vi "Remove Name-UserEvent.vi"(10 "Name":string, 11 "UserEventTimer in":refnum<class "TimerEngine.lvclass">) -> (3 "UserEventTimer out":refnum<class "TimerEngine.lvclass">)   [LabVIEW 2017, in "TimerEngine.lvlib" / "TimerEngine.lvclass"]
uses:
  TimerEngine.lvclass
  TimerEngine.lvclass/TimerEngine.ctl
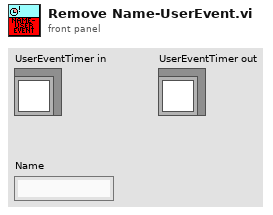
[diagram p1: front panel]
types:
  T1 = typedef "TimerEngine.lvlib/TimerEngine.lvclass/Timer-Userevent.ctl" = refnum<user-event>
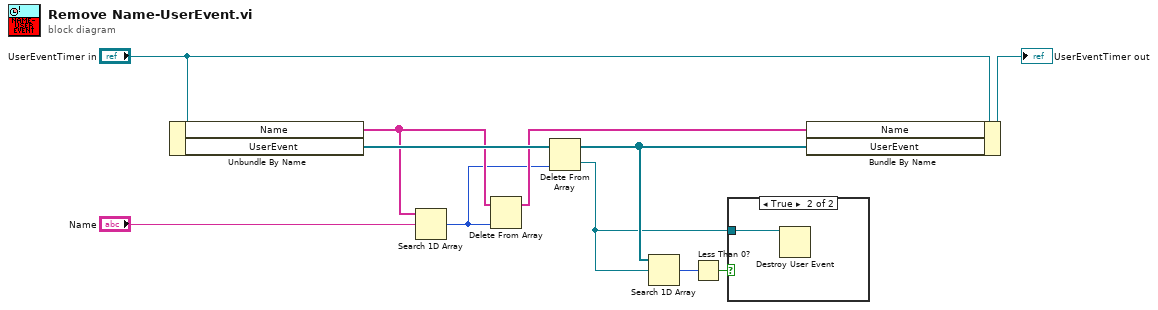
[diagram p0: block diagram]
diagram:
  n1 = Unbundle By Name("UserEventTimer in") -> ("Name"=w7:string[], "UserEvent"=w9:T1[])
  n2 = Search 1D Array(1D array=w7, element="Name") -> (index of element=w5:i32)  [unwired: 1 in]
  n3 = Delete From Array(array=w7, index=w5) -> (array with subset deleted=w6:string[])  [unwired: 1 in, 1 out]
  n4 = Delete From Array(array=w9, index=w5) -> (deleted portion=w2:T1, array with subset deleted=w4:T1[])  [unwired: 1 in]
  n5 = Search 1D Array(1D array=w4, element=w2) -> (index of element=w3:i32)  [unwired: 1 in]
  n6 = Less Than 0?(x=w3) -> (x < 0?=w1:bool)
  n7 = case shown="True" w1 {
    tunnel: w2 -> [_ w12]
    frame False {
    }
    frame True {
      n8 = Destroy User Event(user event=w12) -> ()  [unwired: 1 in, 1 out]
    }
  }
  n9 = Bundle By Name(cluster="UserEventTimer in", "Name"=w6, "UserEvent"=w4) -> (→"UserEventTimer out":refnum<class "TimerEngine.lvclass">)
